vi "Send Response.vi"(0 "reference in":refnum<class "CR slave.lvclass">, 1 "response":string, 2 "data":variant, 5 "error in (no error)":errorcluster) -> (14 "reference out":refnum<class "CR slave.lvclass">, 19 "error out":errorcluster)   [LabVIEW 2019, in "CommandResponse communication.lvlib" / "CR slave.lvclass"]
doc: "Sends response message to master. Should be called after recieving and processing command"
uses:
  CR slave.lvclass
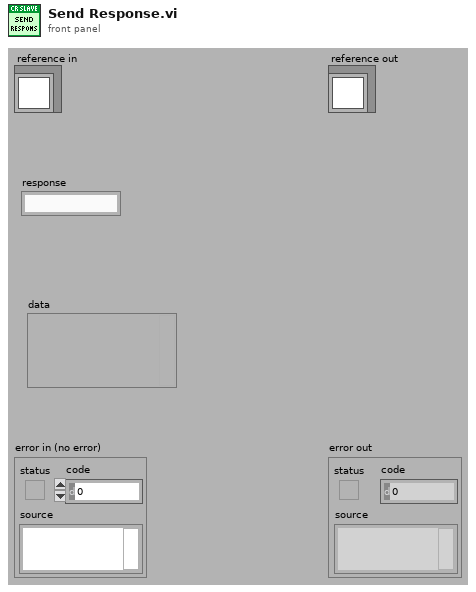
[diagram p1: front panel]
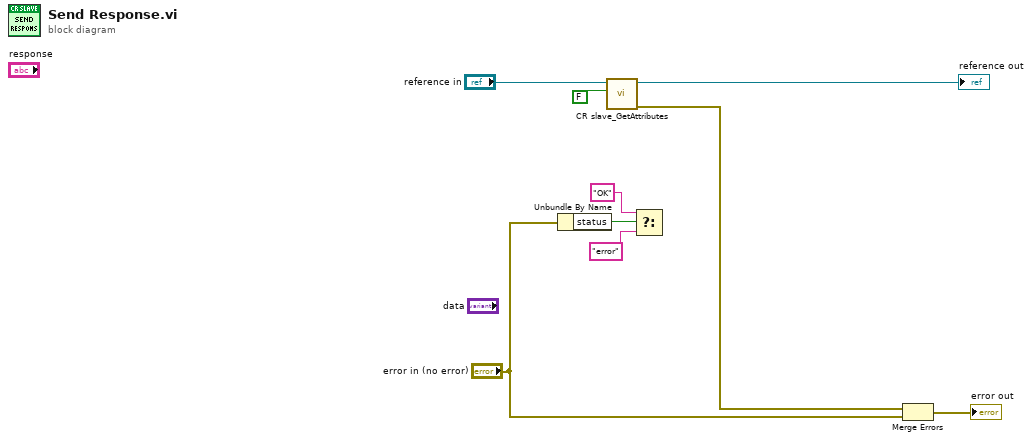
[diagram p0: block diagram]
diagram:
  n1 = Unbundle By Name("error in (no error)") -> ("status"=w3:bool)
  n2 = call "CR slave_GetAttributes.vi"("return data? (T)"=FALSE, "reference in"="reference in") -> ("error out"=w5:errorcluster, "reference out"=→"reference out":refnum<class "CR slave.lvclass">)  [unwired: 6 in, 2 out]
  n3 = Select(t="OK", s=w3, f="error") -> ()  [unwired: 1 out]
  n4 = Merge Errors(w5, "error in (no error)") -> (→"error out":errorcluster)
